vi "Set Hi Press.vi"(7 "init":bool, 8 "error in (no error)":errorcluster, 11 "Stand in":refnum<class "Stand.lvclass">) -> (0 "error out":errorcluster, 2 "Done":bool)   [LabVIEW 2019, in "Stand.lvclass"]
uses:
  Stand.lvclass
  D:/GIT H4000/H4000/src/Device_class/Device.lvclass
  Stand.lvclass/Stand.ctl
  Valve Mode.ctl
  Device_class/Device.lvclass/Device.ctl
  AI_class/AI.lvclass/AI.ctl
  AnalogComparator_class/AnalogComparator.lvclass/AnalogComparator.ctl
  29706e3b-acf2-4be0-8e3a-420f003c1de5.vi
  subvis/FastForward.vi
  AI_class/Get_Values.vi
  Get U max Haskel.vi
  Get Accuracy.vi
  Valve State Mode.vi
  AnalogComparator_class/GetStatus.vi
  Valve State Mode.vi/810e184e-eeb6-4027-a8ae-1422f3ce3d45.vi
  Valve State Mode.vi/57bd4a65-f3dc-44f5-8d68-677c2a197570.vi
  Valve State Mode.vi/03b2f9e4-fceb-4725-9b90-3fd10082a088.vi
  Valve State Mode.vi/2785bab5-dd59-4d13-b638-b9157202fa4a.vi
  Valve State Mode.vi/50faa4b8-a9b4-4cc6-ab66-55c42b424fcd.vi
  Valve State Mode.vi/c882c3fe-b7a7-4419-8f9b-6788aa23338b.vi
  Valve State Mode.vi/3d0d09bd-48e8-482f-b1e2-a36b2bb65234.vi
  Valve State Mode.vi/33d3f26a-dc4a-4f56-bf0a-61d04c5d7434.vi
  Valve State Mode.vi/52af9d47-24d1-4057-80bf-8d93bfb3d17d.vi
  Valve State Mode.vi/bbc9916c-129f-4456-975e-9c3ae3d5db66.vi
  Valve State Mode.vi/a6106d78-2bf9-477e-b655-d47fad07ddfe.vi
  Valve State Mode.vi/e2916439-03c6-4471-bb40-42242a636e27.vi
  Valve State Mode.vi/094228cb-a119-423c-9af8-5a16f059a318.vi
  Valve State Mode.vi/bf5ad1e6-a0ae-4579-ad74-ca8f304cb7cf.vi
  Valve State Mode.vi/eb4d2b76-f0f0-4e1d-bda0-609c5f37b4e7.vi
  Const All Valve.vi
  Global/Global Constant.vi
  <vilib>/addons/_JKI.lib/FPGA_Basic_Components/Counter JKI_FPGA.vi
  <vilib>/addons/_JKI.lib/FPGA_Basic_Components/Counter_32bit JKI_FPGA.vi
  FPGA_API_class/FPGA API.lvclass
  Device_class/Device.lvclass
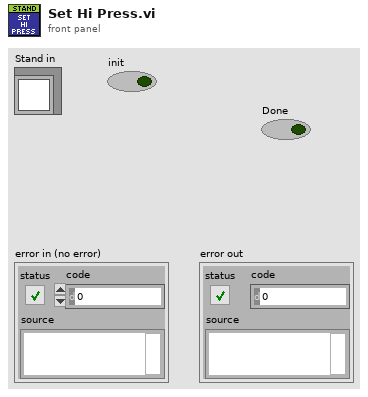
[diagram p1: front panel]
types:
  T1 = typedef "Direction.ctl" = enum8{"DUT", "Chamber"}
  T2 = typedef "Valve Mode.ctl" = enum16{"Filling DUT", "Filling Chamber", "Pump Pressure DUT", "Pump Pressure Chamber", "Haskel Pressure DUT", "Haskel Pressure Chamber", "Slow Release DUT", "Slow Release Chamber", "Fast Release DUT", "Fast Release Chamber", "Fast Release DUT and Chamber", "Leak Pressure DUT", "Leak Pressure Chamber", "Back Pressure DUT", "Back Pressure Chamber", "Fully Closed", "Drain", "Block DUT", "Block Chamber", "filling dut down", "filling chamber down"}
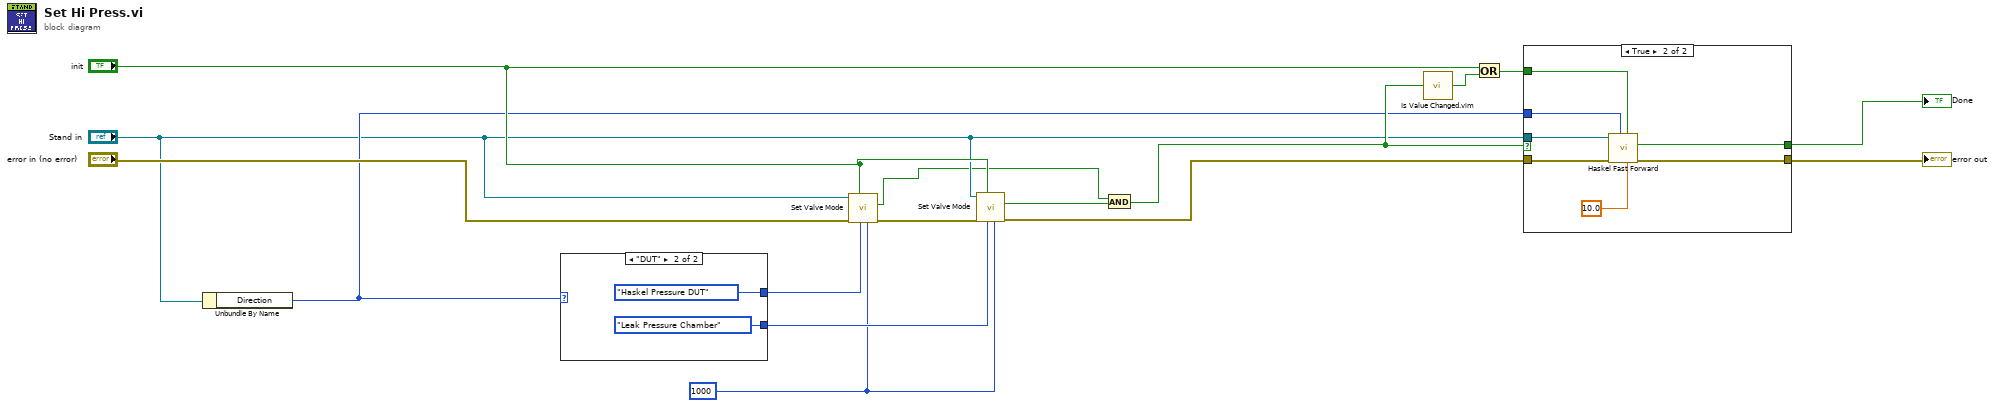
[diagram p0: block diagram]
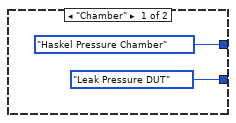
[diagram p2: hidden frame]
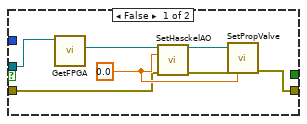
[diagram p3: hidden frame]
diagram:
  w3 = u32 1000 ("time after close")
  n1 = Unbundle By Name("Stand in") -> ("Direction"=w8:T1)
  n2 = case shown="\"DUT\"" w8 {
    tunnel: [Valve_Mode."Haskel Pressure Chamber" ("Valve DIR") Valve_Mode."Haskel Pressure DUT" ("Valve DIR")] -> w6
    tunnel: [Valve_Mode."Leak Pressure DUT" ("Valve DIR") Valve_Mode."Leak Pressure Chamber" ("Valve DIR")] -> w4
    frame "Chamber" {
    }
    frame "DUT" {
    }
  }
  n3 = call "Set Valve Mode.vi"("time after close"=w3, "Valve DIR"=w6, "init"="init", "error in (no error)"="error in (no error)", "Stand in"="Stand in") -> ("error out"=w5:errorcluster, "Done"=w1:bool)  [unwired: 5 in]
  n4 = call "Set Valve Mode.vi"("time after close"=w3, "Valve DIR"=w4, "init"="init", "error in (no error)"=w5, "Stand in"="Stand in") -> ("error out"=w10:errorcluster, "Done"=w2:bool)  [unwired: 5 in]
  n5 = And(x=w1, y=w2) -> (x .and. y?=w12:bool)
  n6 = call "Is Value Changed.vim"("value"=w12) -> ("changed or first call?"=w13:bool)
  n7 = Or(x="init", y=w13) -> (x .or. y?=w14:bool)
  n8 = case shown="True" w12 {
    tunnel: "Stand in" -> [w24 w34]
    tunnel: w10 -> [w22 w33]
    tunnel: [w21 w32] -> w16
    tunnel: w14 -> [_ w31]
    tunnel: [_ w30] -> w15
    tunnel: w8 -> [_ w28]
    frame False {
      w23 = 0.0 ("Haskel in")
      n9 = call "GetFPGA.vi"("Device in"=w24) -> ("FPGA API.lvclass"=w25:refnum<class "FPGA API.lvclass">)  [unwired: 10 in]
      n10 = call-dynamic "SetHasckelAO.vi"("FPGA API in"=w25, "Haskel in"=w23, "error in (no error)"=w22) -> ("FPGA API out"=w27:refnum<class "FPGA API.lvclass">, "error out"=w26:errorcluster)  [unwired: 11 in]
      n11 = call-dynamic "SetPropValve.vi"("FPGA API in"=w27, "error in (no error)"=w26, "AO 1"=w23) -> ("error out"=w21:errorcluster)  [unwired: 11 in, 1 out]
    }
    frame True {
      n12 = call "Haskel Fast Forward.vi"("Time Target (s)"=10.0, "Init"=w31, "Direction"=w28, "error in (no error)"=w33, "Stand in"=w34) -> ("error out"=w32:errorcluster, "Done"=w30:bool)  [unwired: 5 in]
    }
  }
  "error out" <- w16
  "Done" <- w15
